vi "Write Interlock_Enable.vi"(8 "error in":errorcluster, 10 "INTLK_Enable":bool, 11 "6700C in":refnum<class "6700C.lvclass">) -> (0 "error out":errorcluster, 3 "6700C out":refnum<class "6700C.lvclass">)   [LabVIEW 2019, in "6700C.lvlib" / "6700C.lvclass"]
uses:
  Library/6700C.lvclass
  C:/Users/Public/Documents/Development/builds/Engine/Monitored Actor.lvlibp/Monitored Actor/Monitored Actor/Monitored Actor.lvclass
  builds/Engine/Monitored Actor.lvlibp/Monitored Actor/Monitored Actor/Read Actor Label.vi
  builds/Instruments/PowerSupply.lvlibp/Library/PowerSupply.lvclass
  <vilib>/ErrorRing/Error Ring.xnode
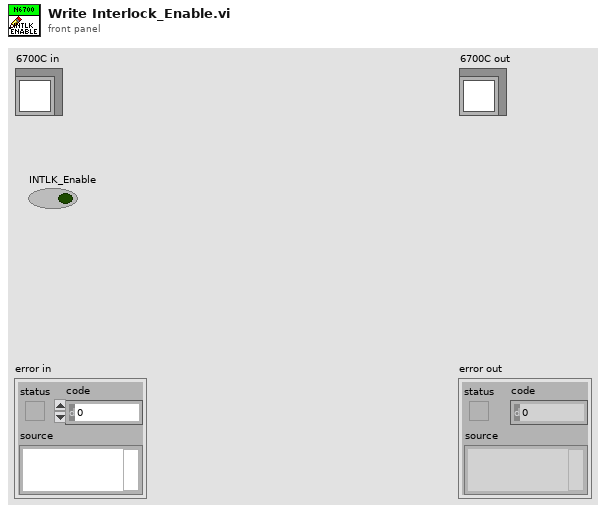
[diagram p1: front panel]
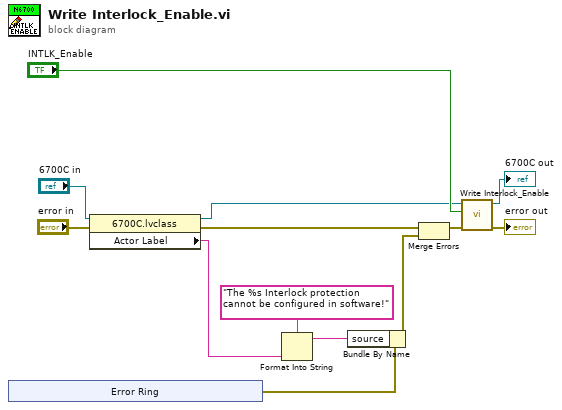
[diagram p0: block diagram]
diagram:
  n1 = xnode "Error Ring"() -> ("error out"=w7:errorcluster)
  n2 = property class="6700C.lvclass"(reference="6700C in", error in="error in") -> (reference out=w2:refnum<class "6700C.lvclass">, error out=w9:errorcluster, "Actor Label"=w8:string)
  n3 = Format Into String(format string="The %s Interlock protection cannot be configured in software!", w8) -> (resulting string=w6:string)  [unwired: 2 in, 1 out]
  n4 = Bundle By Name(cluster=w7, "source"=w6) -> (w10:errorcluster)
  n5 = Merge Errors(w9, w10) -> (w1:errorcluster)
  n6 = call-parent "Write Interlock_Enable.vi"("error in"=w1, "INTLK_Enable"="INTLK_Enable", "PowerSupply in"=w2) -> ("error out"=→"error out":errorcluster, "PowerSupply out"=→"6700C out":refnum<class "6700C.lvclass">)  [unwired: 7 in]
